vi "Robot Global.vi"() -> ()   [LabVIEW 2013]
uses:
  <vilib>/ActorFramework/Message Enqueuer/Message Enqueuer.lvclass
panel:
  out "Drive Train Queue":refnum<class "Message Enqueuer.lvclass">
  out "Robot Queue":refnum<class "Message Enqueuer.lvclass">
  out "Driver Queue":refnum<class "Message Enqueuer.lvclass">
  out "Driver XBox Controller Queue":refnum<class "Message Enqueuer.lvclass">
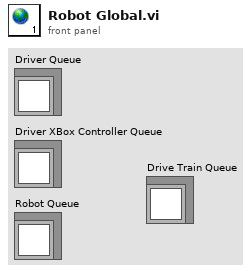
[diagram p1: front panel]
diagram:
